vi "204_SubscribePoll_StreamingNode.vi"() -> ()   [LabVIEW 2009]
uses:
  <instrlib>/Zurich Instruments LabOne/Public/Data/ziTypeDemodSampleEx.ctl
  <instrlib>/Zurich Instruments LabOne/Public/Data/ziTypeDemodVectorEx.ctl
  <instrlib>/Zurich Instruments LabOne/Public/Configure/ziGetValueString.vi
  <instrlib>/Zurich Instruments LabOne/Public/Data/ziGetEventDemodSample.vi
  <instrlib>/Zurich Instruments LabOne/Public/Data/ziGetEventDemodVector.vi
  <instrlib>/Zurich Instruments LabOne/Zurich Instruments LabOne.lvlib
panel:
  out "Instrument Type":string
  out "Waveform Chart":dbl[](graph)
  in  "stop":bool
  out "Connected?":bool
  out "Error Out":errorcluster
  in  "Address":string="DEV"
  out "Tab Control":T1(tab)
  out "Demod Sample Out":T2 {"Aux In 1 (V)" format="%#_5p"; "Aux In 0 (V)" format="%#_5p"; "X (Vrms)" format="%#_5p"; "Y (Vrms)" format="%#_5p"; "Osc Phase (rad)" format="%#.3g"}
  out "Demod Vector out":T3
  # "Subscribe and Poll \nStreaming Node \nThis VI shows how to capture the data from a streaming node using subscribe and poll commands. In this example we will use a demodulator node.\n\nThe demod node is a streaming node that returns output samples of the demodulator. This streaming concept allows high data transfer rates, which cannot be achieved with the get command.\n\nIn comparison to the LabOne user interface:\n- the \"Demod Sample Out\" cluster behaves similar to the Numeric tab\n- the waveform that is wired to show R behaves similarly to the Plotter tab.\n \nSee block diagram for the VI description.\n\nRequirements: Any Zurich Instrument lock-in amplifier\n\nTo run\n1- Type the Instrument ID \n2- Run the VI\n3- Do the test described on the right \n\nTested Devices:\n- HF2LI\n- UHFLI\n- MFLI\n- GHFLI\n- SHFLI\n\n(c) Zurich Instruments.  ALL RIGHTS RESERVED."
  # "Test the impact of changing the data transfer settings on the LabOne graphical user interface (GUI) \n1- Run the VI. \n     Note that this VI subscribes to the first demodulator of the Lock-in amplifier. You can change it in the back panel if you like (step 2).  \n2- On the LabOne GUI change the data transfer settings highlighted below by the red rectangle and observe how the indicators above updates:\n    2.1 Start the GUI on default settings\n    2.2 set the data transfer rate to 1 s  (the update rate of the indicators slow)\n    2.3 set the data transfer rate to 1 ks (fast update)\n    2.4 Turn off the data transfer rate (no update until turned on)\nNote that the data transfer settings can also be updated using the ziSetValue command (see 202)"
  # "The Lock-in panel of your instrument might slightly differ depending on the instrument \nand installed options"
  # "This instrument type streams the data as individual samples per timestamps. LabOne's LabVIEW API parses these samples to individual arrays of the samples' content to make them easier to work with."
  # "This instrument type streams the data as vectors of a burst of samples. LabOne's LabVIEW API parses these vectors to individual arrays of its content to make them easier to work with."
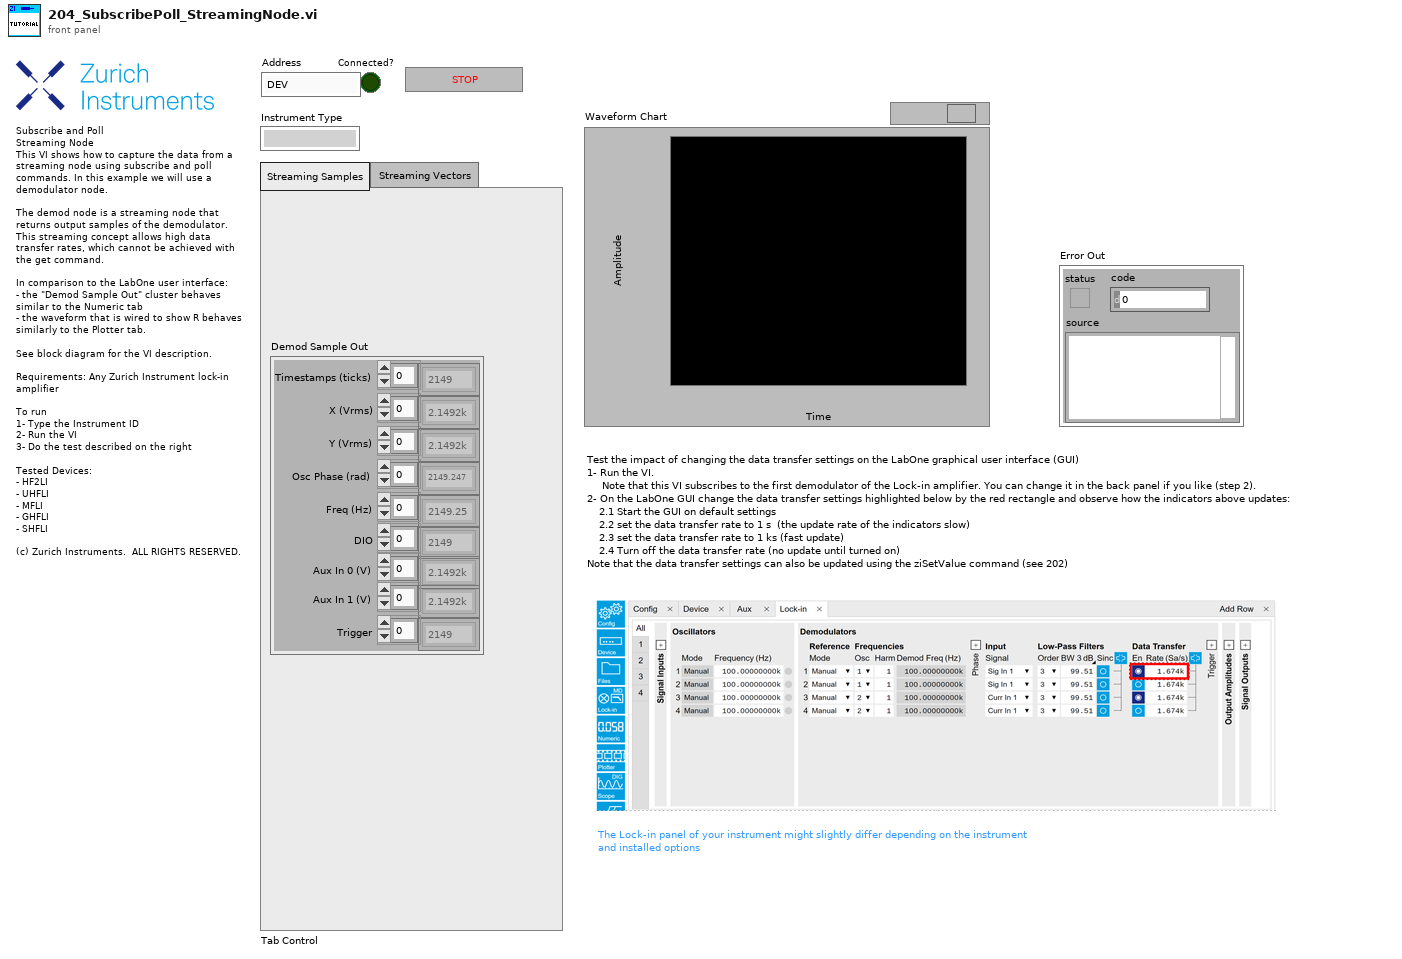
[diagram p1: front panel]
types:
  T1 = enum32{"Streaming Samples", "Streaming Vectors "}
  T2 = typedef "Zurich Instruments LabOne.lvlib/ziTypeDemodSampleEx.ctl" = cluster{"Timestamps (ticks)":u64[], "X (Vrms)":dbl[], "Y (Vrms)":dbl[], "Osc Phase (rad)":dbl[], "Freq (Hz)":dbl[], "DIO":u32[], "Aux In 0 (V)":dbl[], "Aux In 1 (V)":dbl[], "Trigger":u32[]}
  T3 = typedef "Zurich Instruments LabOne.lvlib/ziTypeDemodVectorEx.ctl" = cluster{"Timestamps (ticks)":u64[], "X (Vrms)":dbl[], "Y (Vrms)":dbl[], "triggersource":u8[], "burstlength":u32[], "burstoffset":u32[], "triggerindex":u32[], "triggertimestamps":u64[], "centerfreq":dbl[], "rfpath":u8[], "oscillatorsource":u16[], "harmonic":u16[], "signalsource":u16[], "oscillatorfreq":dbl[]}
  T4 = typedef "Zurich Instruments LabOne.lvlib/ziTypeHandle.ctl" = cluster{"handleValid":bool, "Conn":u64, "Path Prefix":string, "Handle":u64, "Connected":bool, "Clockbase(s)":dbl}
  T5 = typedef "Zurich Instruments LabOne.lvlib/ziTypePollType.ctl" = enum16{"NONE", "DOUBLE_DATA", "INTEGER_DATA", "DEMOD_SAMPLE", "SCOPE_WAVE_HF2", "AUXIN_SAMPLE", "DIO_SAMPLE", "BYTE_ARRAY", "PWA_WAVE", "9", "10", "11", "12", "13", "14", "15", "TREE_CHANGE_DEPRI", "17", "ERROR", "19", "20", "21", "22", "23", "24", "25", "26", "27", "28", "29", "30", "31", "DOUBLE_DATA_TS", "INTEGER_DATA_TS", "34", "SCOPE_WAVE", "SCOPE_WAVE_EX", "37", "BYTE_ARRAY_TS", "39", "40", "41", "42", "43", "44", "45", "CNT_DATA", "47", "TREE_CHANGE", "49", "50", "51", "52", "53", "54", "55", "56", "57", "58", "59", "60", "61", "62", "63", "SWEEPER_DATA", "SPECTRUM_DATA", "ADVISOR_DATA", "VECTOR_DATA", "IMP_DATA", "SHF_GENERATOR_WAVEFORM_DATA", "SHF_RESULT_LOGGER_DATA", "SHF_SCOPE_DATA", "DEMOD_VECTOR"}
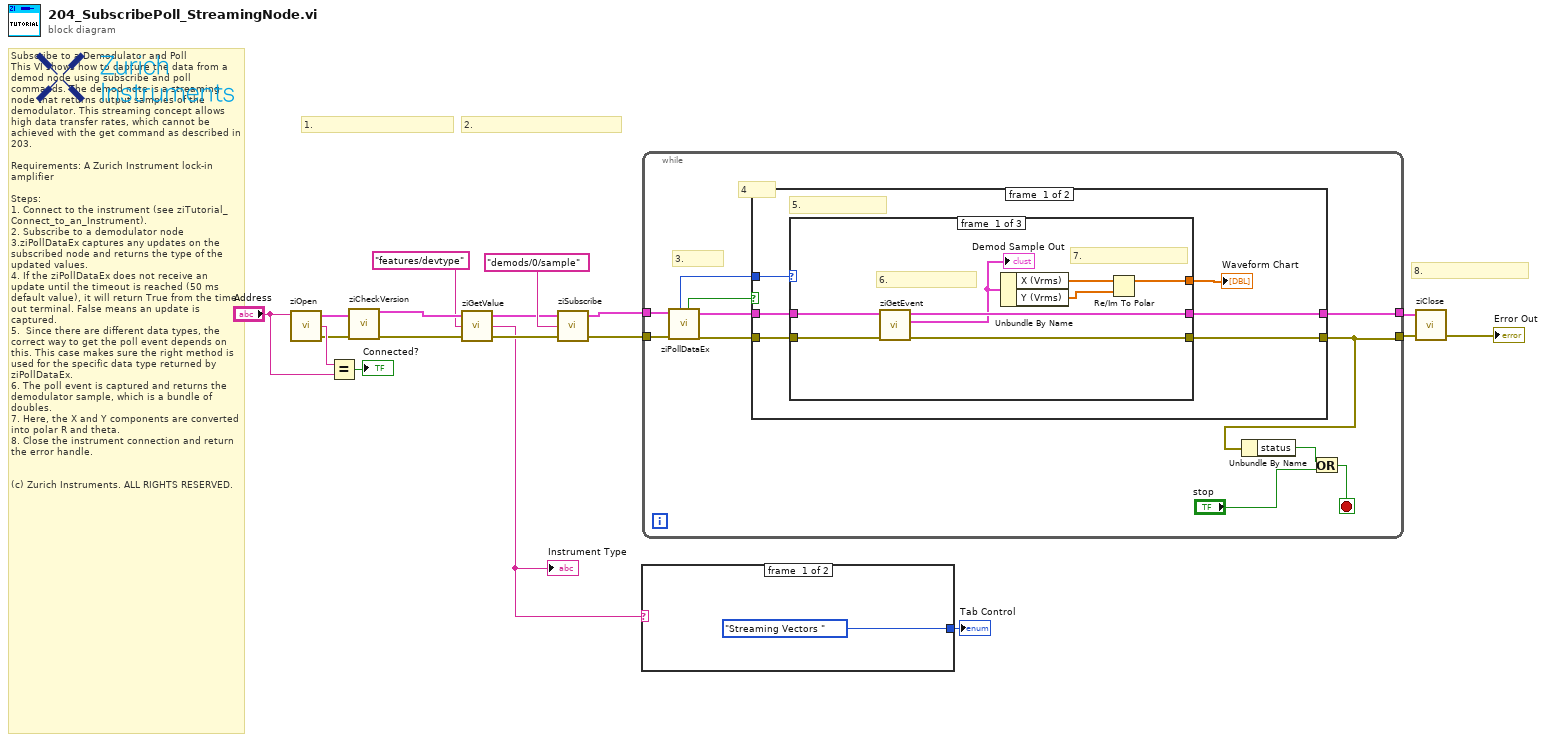
[diagram p0: block diagram]
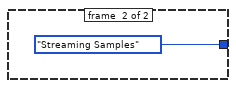
[diagram p2: hidden frame]
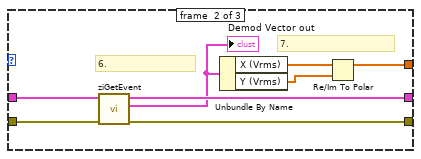
[diagram p3: hidden frame]
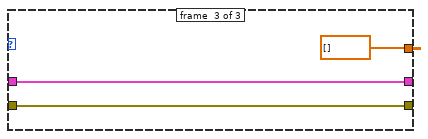
[diagram p4: hidden frame]
diagram:
  # "2."
  # "1."
  # "8."
  # "Subscribe to a Demodulator and Poll\nThis VI shows how to capture the data from a demod node using subscribe and poll commands. The demod note is a streaming node that returns output samples of the demodulator. This streaming concept allows high data transfer rates, which cannot be achieved with the get command as described in 203. \n\nRequirements: A Zurich Instrument lock-in amplifier\n\nSteps:\n1. Connect to the instrument (see ziTutorial_Connect_to_an_Instrument).\n2. Subscribe to a demodulator node \n3.ziPollDataEx captures any updates on the subscribed node and returns the type of the updated values. \n4. If the ziPollDataEx does not receive an update until the timeout is reached (50 ms default value), it will return True from the time out terminal. False means an update is captured.\n5.  Since there are different data types, the correct way to get the poll event depends on this. This case makes sure the right method is used for the specific data type returned by ziPollDataEx. \n6. The poll event is captured and returns the demodulator sample, which is a bundle of doubles.\n7. Here, the X and Y components are converted into polar R and theta. \n8. Close the instrument connection and return the error handle.\n\n\n(c) Zurich Instruments. ALL RIGHTS RESERVED."
  n1 = call <instrlib>:"ziOpen.vi"("Address"="Address") -> ("Error Out"=w13:errorcluster, "Selected Device"=w16:string, "HandleOut"=w14:T4)  [unwired: 1 in, 2 out]
  n2 = Equal?(x=w16, y="Address") -> (x = y?=→"Connected?":bool)
  n3 = call <instrlib>:"ziCheckVersion.vi"("Handle In"=w14, "Error In"=w13) -> ("Handle Out"=w7:T4, "Error Out"=w5:errorcluster)  [unwired: 11 in, 1 out]
  n4 = call-poly <instrlib>:"ziGetValue.vi"("error in"=w5, "Path"="features/devtype", "Handle In"=w7) -> ("error out"=w4:errorcluster, "Value"=w1:string, "Handle Out"=w6:T4)
  "Instrument Type" <- w1
  n5 = call <instrlib>:"ziSubscribe.vi"("error in"=w4, "Path ()"="demods/0/sample" ("path"), "Handle In"=w6) -> ("error out"=w11:errorcluster, "Handle Out"=w10:T4)  [unwired: 1 in]
  n6 = case shown="\"HF2IS\", \"HF2LI\", \"MFIA\", \"MFLI\", \"UHFLI\", Default" w1 {
    tunnel: [T1."Streaming Vectors " ("Tab Control 2") T1."Streaming Samples" ("Tab Control 2")] -> w2
    frame #0 {
    }
    frame #1 {
    }
  }
  "Tab Control" <- w2
  n7 = while {
    tunnel: w11 -> [w29]
    tunnel: w10 -> [w30]
    tunnel: [w31] -> w9
    tunnel: [w21] -> w8
    stop <- w22 stop-if-true
    # "3."
    # "4"
    n8 = call <instrlib>:"ziPollDataEx.vi"("error in"=w29, "Handle In"=w30) -> ("error out"=w27:errorcluster, "Handle Out"=w28:T4, "Timed Out"=w26:bool, "ziValueType"=w25:T5)  [unwired: 2 in, 4 out]
    n9 = case shown="False" w26 {
      tunnel: [w37 w58] -> w31
      tunnel: [w36 w57] -> w21
      tunnel: w28 -> [w35 w58]
      tunnel: w27 -> [w34 w57]
      tunnel: w25 -> [w33 _]
      frame #0 {
        # "5."
        n10 = case shown="\"DEMOD_VECTOR\"" w33 {
          tunnel: [w45 w53 w56] -> w37
          tunnel: [w44 w52 w55] -> w36
          tunnel: w35 -> [w43 w51 w56]
          tunnel: w34 -> [w42 w50 w55]
          tunnel: [w38 w46 dbl[] []] -> w32
          frame #0 {
            # "7."
            # "6."
            n11 = call-poly <instrlib>:"ziGetEvent.vi"("Error In"=w42, "Handle In"=w43) -> ("Error Out"=w44:errorcluster, "Demod Sample Out"=w41:T2, "Handle Out"=w45:T4)  [unwired: 7 in]
            "Demod Sample Out" <- w41
            n12 = Unbundle By Name(w41) -> ("X (Vrms)"=w40:dbl[], "Y (Vrms)"=w39:dbl[])
            n13 = Re/Im To Polar(2:w39, 3:w40) -> (1:w38:dbl[])  [unwired: 1 out]
          }
          frame #1 {
            # "7."
            # "6."
            n14 = call-poly <instrlib>:"ziGetEvent.vi"("Error In"=w50, "Handle In"=w51) -> ("Error Out"=w52:errorcluster, "Demod Vector Out"=w49:T3, "Handle Out"=w53:T4)  [unwired: 7 in]
            "Demod Vector out" <- w49
            n15 = Unbundle By Name(w49) -> ("X (Vrms)"=w48:dbl[], "Y (Vrms)"=w47:dbl[])
            n16 = Re/Im To Polar(2:w47, 3:w48) -> (1:w46:dbl[])  [unwired: 1 out]
          }
          frame #2 {
          }
        }
        "Waveform Chart" <- w32
      }
      frame #1 {
      }
    }
    n17 = Unbundle By Name(w21) -> ("status"=w23:bool)
    n18 = Or(x=w23, y="stop") -> (x .or. y?=w22:bool)
  }
  n19 = call <instrlib>:"ziClose.vi"("Error In"=w8, "Handle In"=w9) -> ("Error Out"=→"Error Out":errorcluster)  [unwired: 2 in, 1 out]
